vi "Autonomous IndependentAPRIL6TH (1).vi"() -> ()   [LabVIEW 2016]
doc: "This VI is called when autonomous begins, and will automatically be terminated when autonomous ends. You can carry out timed or sensor driven robot movement independently without needing to return to the caller."
uses:
  <vilib>/Rock Robotics/WPI/Utilities/WPI_GetSetVariantRefNum.vi
  <vilib>/Rock Robotics/Network Tables/NT Read String.vi
  <vilib>/Rock Robotics/Network Tables/NT Write Numeric Array.vi
  <vilib>/Rock Robotics/WPI/RobotDrive/WPI_RobotDriveArcadeDrive_Standard(NoSaturation).vi
  <vilib>/Rock Robotics/Network Tables/NT Write Number.vi
  Robot Global Data.vi
  <vilib>/Rock Robotics/WPI/Counter/WPI_CounterDigitalInputToDigitalSource.vi
  <vilib>/Rock Robotics/SystemInterfaces/DIO/FPGA_DIOChannel.ctl
panel:
  out "Hook Center Cons":dbl
  out "gyro":dbl
  out "sonar distance (inches)":dbl
  out "Encoder Loop":dbl
  out "Encoder Loop":string
  out "Current Movement, for debugging 2":T1 {"Y Joystick Value" scale=1.0..-1.0; "X Joystick Value" scale=-1.0..1.0}
  in  "Array of robot movements 2":T2(array[cluster])=[{"X Joystick Value"=0.39393939393939403, "Y Joystick Value"=0.0, "Delay (sec)"=1.0, "Movement Name"="turn"}, {"X Joystick Value"=-0.3737373737373737, "Y Joystick Value"=0.0, "Delay (sec)"=1.0, "Movement Name"="turn back"}] {"Y Joystick Value" scale=1.0..-1.0; "X Joystick Value" scale=-1.0..1.0}
  out "Current Movement, for debugging":T1 {"Y Joystick Value" scale=1.0..-1.0; "X Joystick Value" scale=-1.0..1.0}
  in  "Array of robot movements":T2(array[cluster])=[{"X Joystick Value"=0.39393939393939403, "Y Joystick Value"=0.0, "Delay (sec)"=1.0, "Movement Name"="turn"}, {"X Joystick Value"=-0.3737373737373737, "Y Joystick Value"=0.0, "Delay (sec)"=1.0, "Movement Name"="turn back"}] {"Y Joystick Value" scale=1.0..-1.0; "X Joystick Value" scale=-1.0..1.0}
  # "Sensor Readings\nConstanly updated in\nwhile loopes"
  # "Be sure to right-click and choose Data Operations>>Make Current Value default if you want to save the array values with the VI"
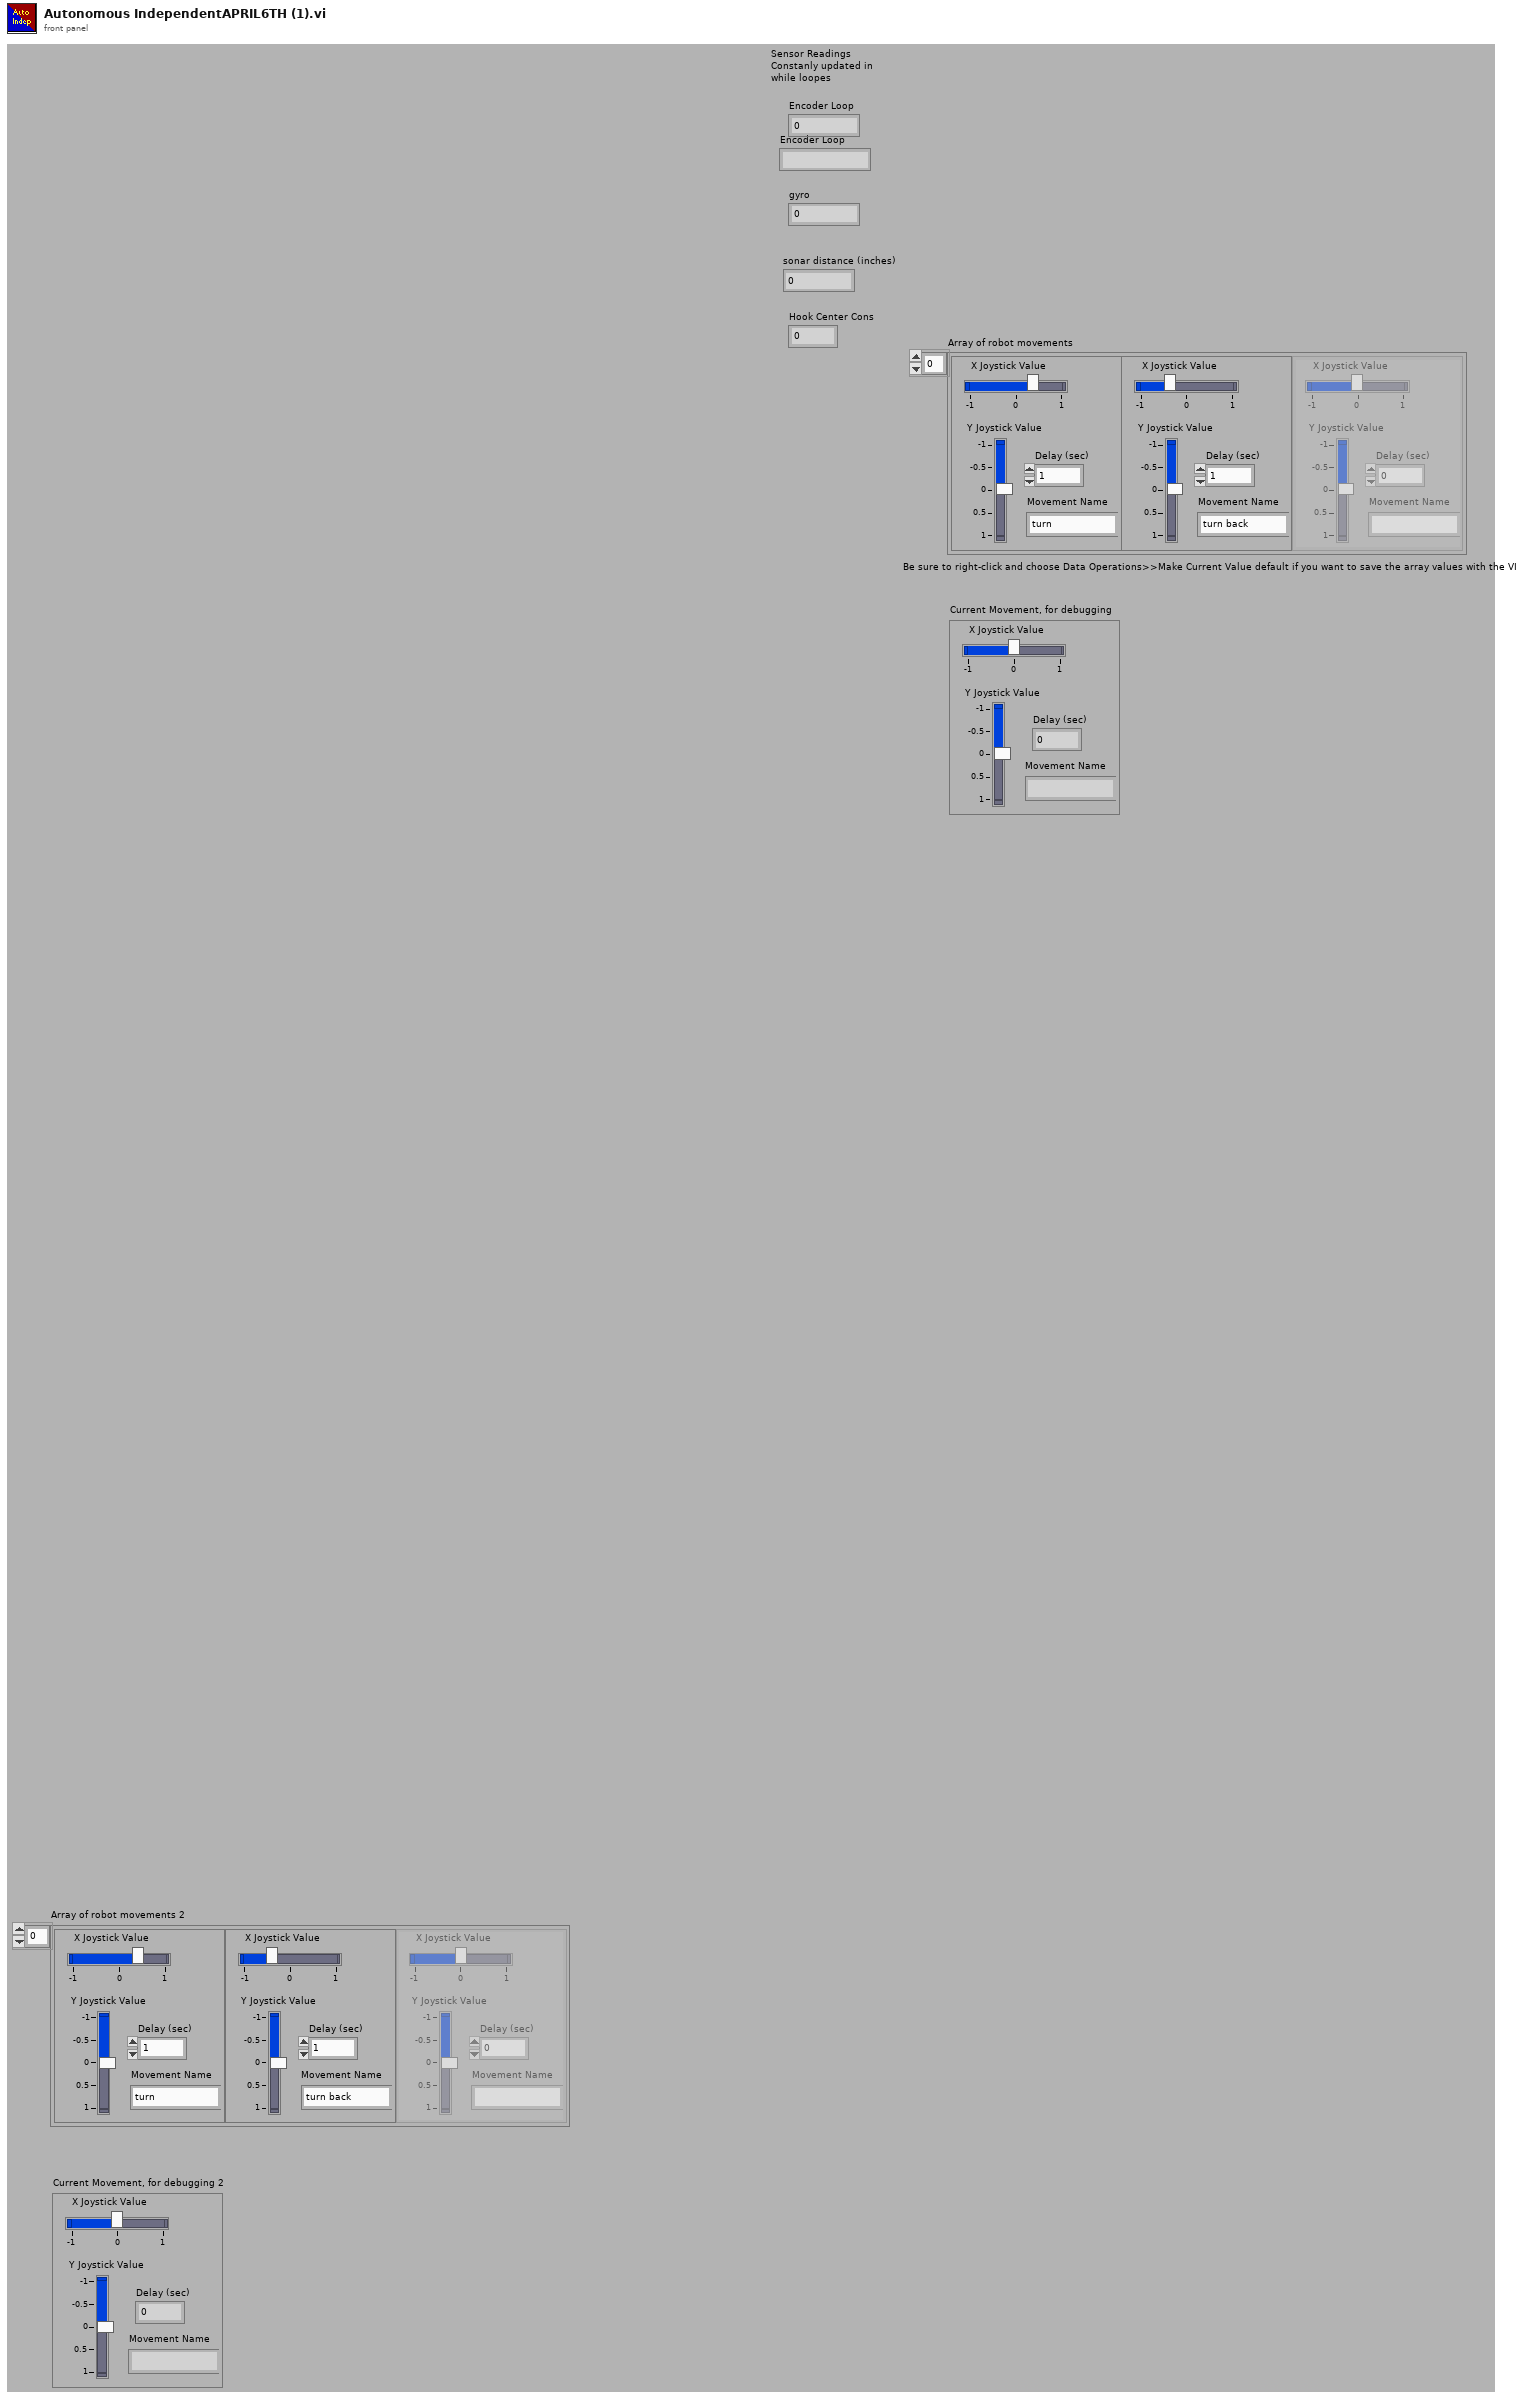
[diagram p1: front panel]
types:
  T1 = cluster{"X Joystick Value":dbl, "Y Joystick Value":dbl, "Delay (sec)":dbl, "Movement Name":string}
  T2 = cluster{"X Joystick Value":dbl, "Y Joystick Value":dbl, "Delay (sec)":dbl, "Movement Name":string}[]
  T3 = typedef "FPGA_DIOChannel.ctl" = enum8{"DIO 0", "DIO 1", "DIO 2", "DIO 3", "DIO 4", "DIO 5", "DIO 6", "DIO 7", "DIO 8", "DIO 9", "DIO MXP 0", "DIO MXP 1", "DIO MXP 2", "DIO MXP 3", "DIO MXP 4", "DIO MXP 5", "DIO MXP 6", "DIO MXP 7", "DIO MXP 8", "DIO MXP 9", "DIO MXP 10", "DIO MXP 11", "DIO MXP 12", "DIO MXP 13", "DIO MXP 14", "DIO MXP 15", "SPI Port CS1", "SPI Port CS2", "SPI Port CS3", "SPI Port MISO", "SPI Port MOSI", "Invalid"}
  T4 = typedef "WPI_DigitalInputDevRef.ctl" = cluster{"DevStatus":errorcluster, "DIO Channel":T3}
  T5 = typedef "FPGA_CounterEncoderSourceConvertionLVSourceType.ctl" = cluster{"DevStatus":errorcluster, "AnalogTriggerMode?":bool, "DigitalMode":cluster{"DIO Channel":T6}, "AnalogTriggerMode":cluster{"AnalogTriggerIndex":T7, "OutputType":T8}}
  T6 = typedef "FPGA_DIODigitalSourceChannel.ctl" = enum8{"DIO 0", "DIO 1", "DIO 2", "DIO 3", "DIO 4", "DIO 5", "DIO 6", "DIO 7", "DIO 8", "DIO 9", "DIO MXP 0", "DIO MXP 1", "DIO MXP 2", "DIO MXP 3", "DIO MXP 4", "DIO MXP 5", "DIO MXP 6", "DIO MXP 7", "DIO MXP 8", "DIO MXP 9", "DIO MXP 10", "DIO MXP 11", "DIO MXP 12", "DIO MXP 13", "DIO MXP 14", "DIO MXP 15", "Disabled"}
  T7 = typedef "FPGA_AnalogTriggerIndex.ctl" = enum8{"Trig 0", "Trig 1", "Trig 2", "Trig 3", "Trig 4", "Trig 5", "Trig 6", "Trig 7", "Invalid"}
  T8 = typedef "FPGA_AnalogTriggerOutType.ctl" = enum16{"InWindow", "TriggerState", "Rising", "Falling"}
  T9 = typedef "WPI_EncoderDevRef.ctl" = cluster{"DevStatus":errorcluster, "EncoderIndex":T10, "CounterIndex":T11, "DistancePerCount":dbl, "Decoding Type":T12}
  T10 = typedef "FPGA_EncoderIdx.ctl" = enum8{"Enc 0", "Enc 1", "Enc 2", "Enc 3", "Enc 4", "Enc 5", "Enc 6", "Enc 7", "Invalid"}
  T11 = typedef "FPGA_CounterCtrSystemIndex.ctl" = enum8{"Ctr 0", "Ctr 1", "Ctr 2", "Ctr 3", "Ctr 4", "Ctr 5", "Ctr 6", "Ctr 7", "Invalid"}
  T12 = typedef "WPI_EncoderType.ctl" = enum16{"1x", "2x", "4x"}
  T13 = typedef "WPI_JoystickDevRef.ctl" = cluster{"Device":T14}
  T14 = typedef "WPI_JoystickDeviceEnum.ctl" = enum16{"USB 0", "USB 1", "USB 2", "USB 3", "USB 4", "USB 5"}
  T15 = typedef "WPI_DriverStationPositionInfo.ctl" = enum16{"1", "2", "3"}
  T16 = typedef "WPI_RobotDriveDevRef.ctl" = cluster{"DevStatus":errorcluster, "Motors[]":T17[], "Square Inputs":bool, "Max Output":dbl}
  T17 = typedef "WPI_MotorControlDeviceRef.ctl" = cluster{"DeviceStatus":errorcluster, "Type":T18, "PWM":cluster{"PWM Channel":T19, "DeadBand":T20}, "CAN":cluster{"Device Number":u8, "SetOutput VI Ref":variant, "GetOutput VI Ref":variant, "Enable VI Ref":variant, "Disable VI Ref":variant, "Data":variant}, "Invert":bool}
  T18 = typedef "WPI_MotorControlType.ctl" = enum16{"PWM", "CAN"}
  T19 = typedef "FPGA_DIOPWMChannel.ctl" = enum8{"PWM 0", "PWM 1", "PWM 2", "PWM 3", "PWM 4", "PWM 5", "PWM 6", "PWM 7", "PWM 8", "PWM 9", "PWM MXP 0", "PWM MXP 1", "PWM MXP 2", "PWM MXP 3", "PWM MXP 4", "PWM MXP 5", "PWM MXP 6", "PWM MXP 7", "PWM MXP 8", "PWM MXP 9", "Invalid"}
  T20 = typedef "WPI_PWMDeadband.ctl" = cluster{"Name":string, "maxPositivePwm":i32, "minPositivePwm":i32, "centerPwm":i32, "maxNegativePwm":i32, "minNegativePwm":i32, "angularRange":u16}
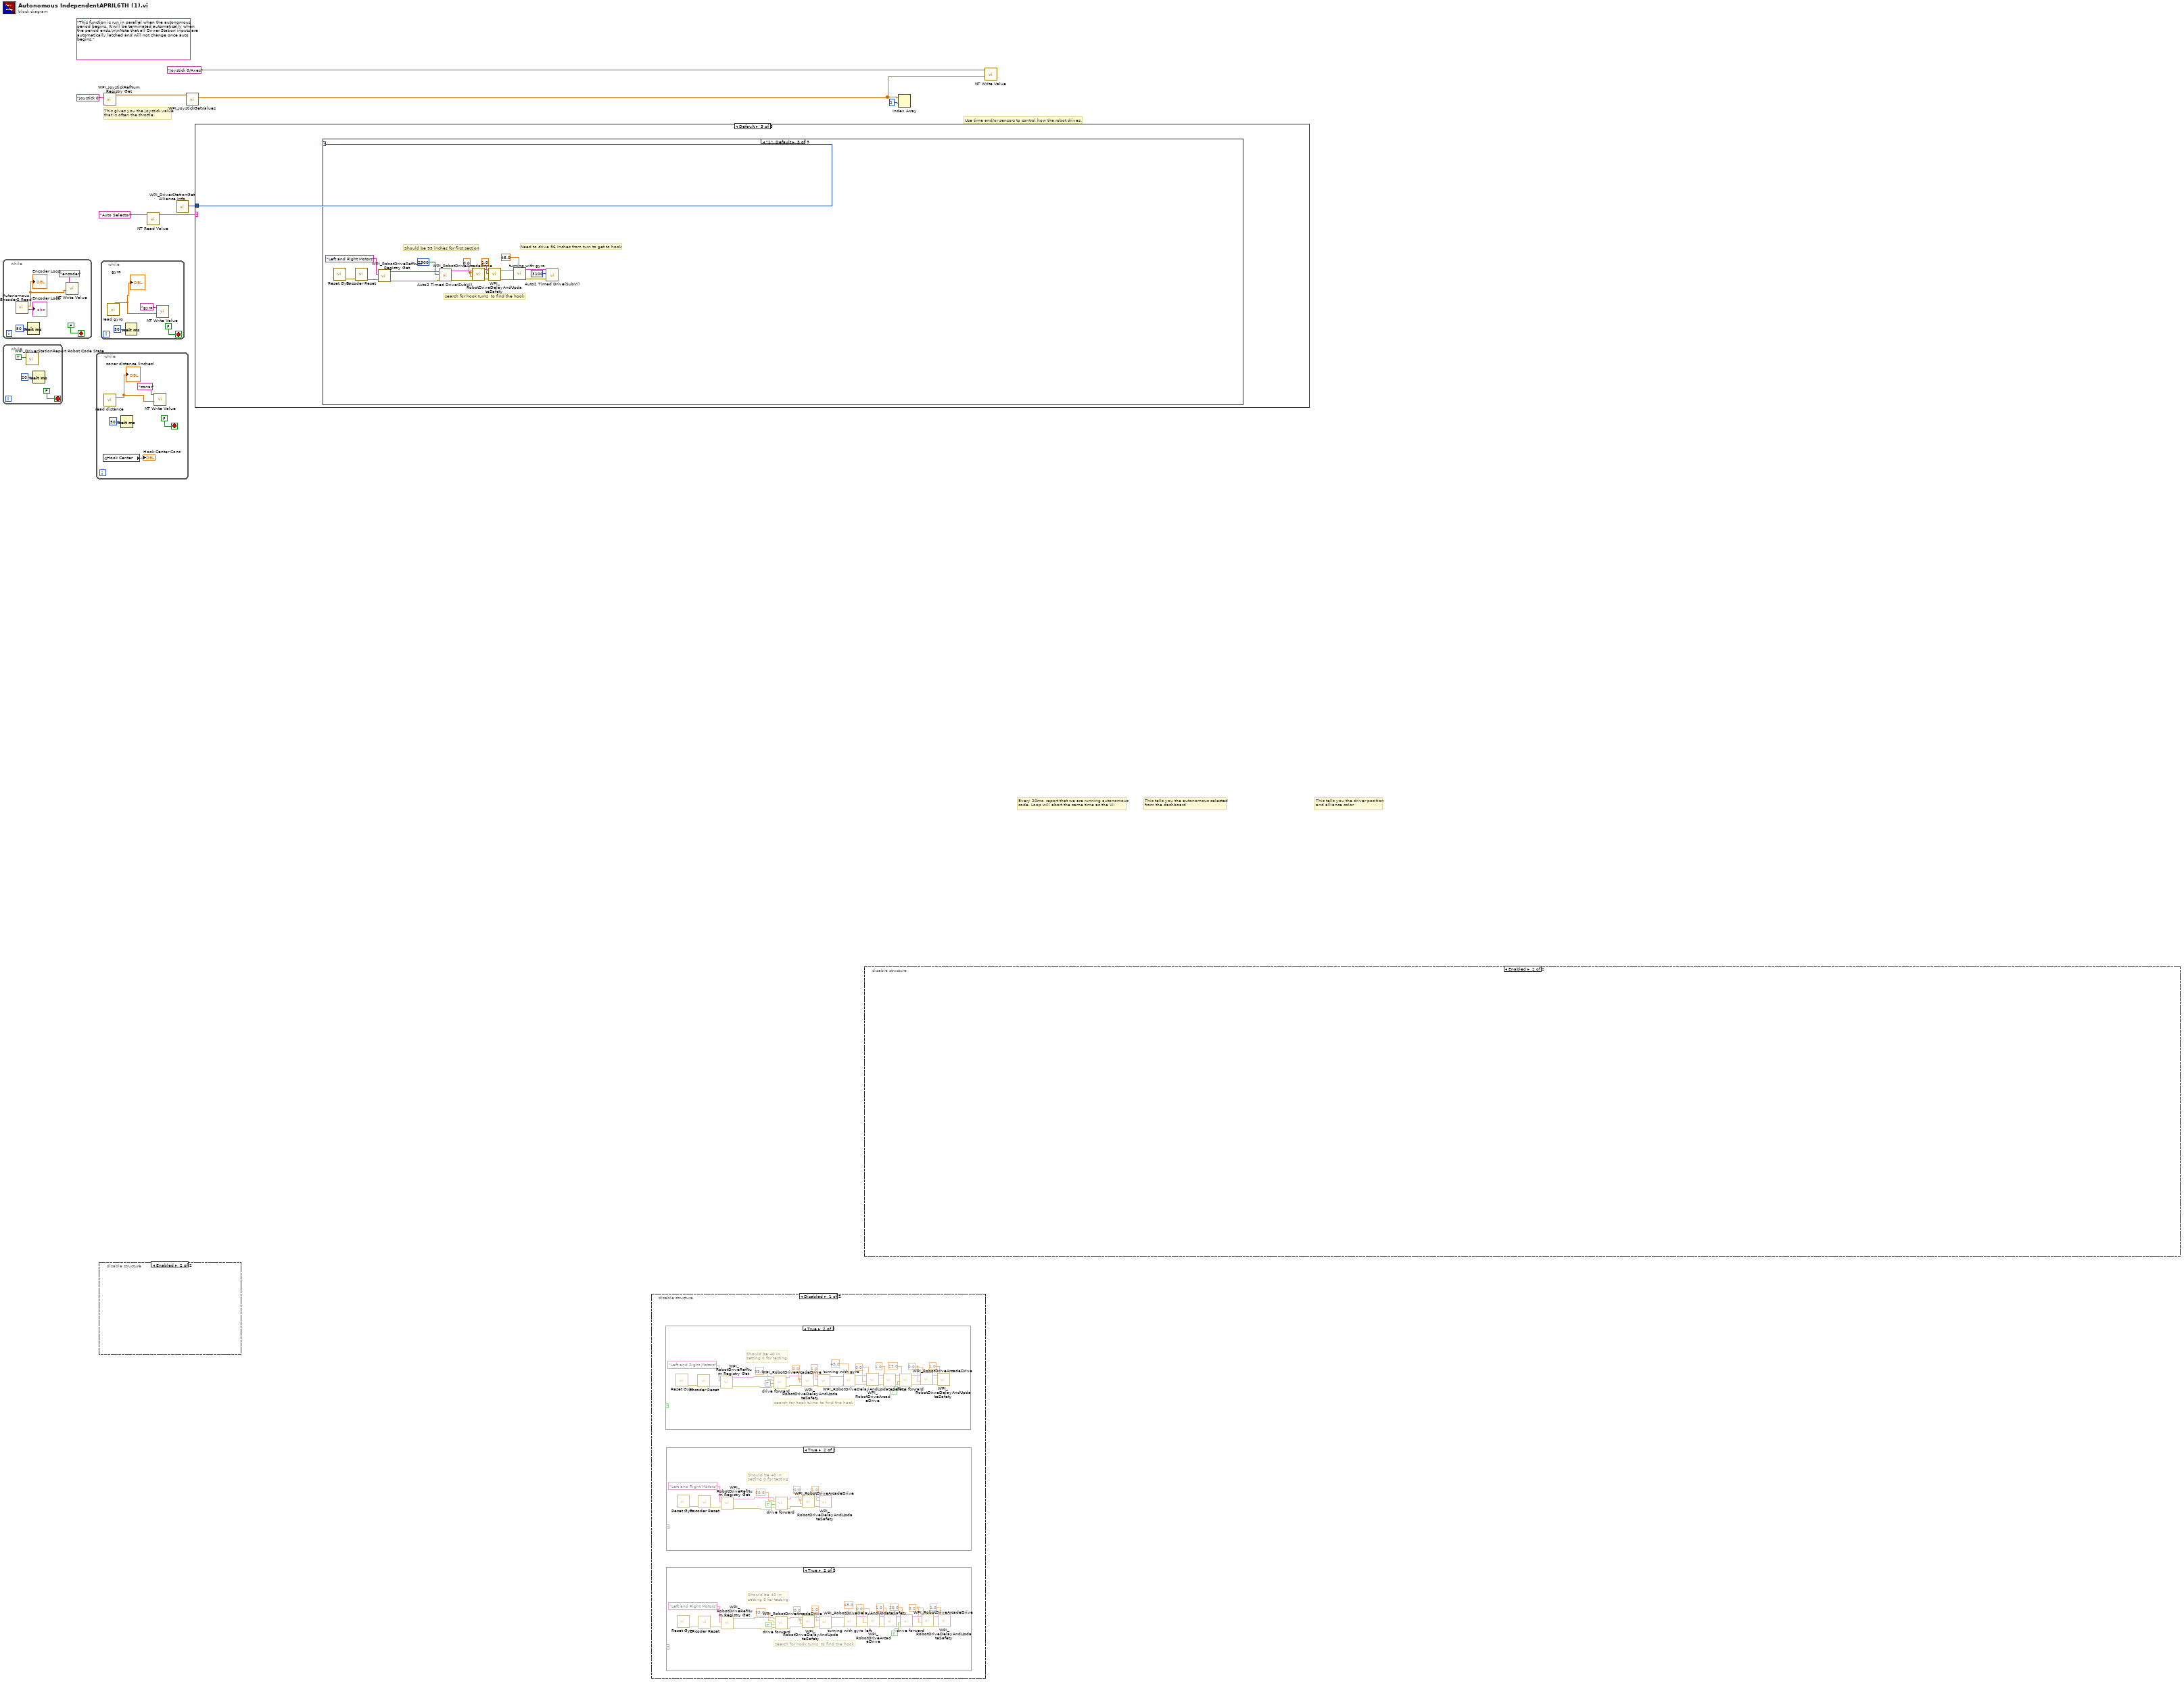
[diagram p0: block diagram]
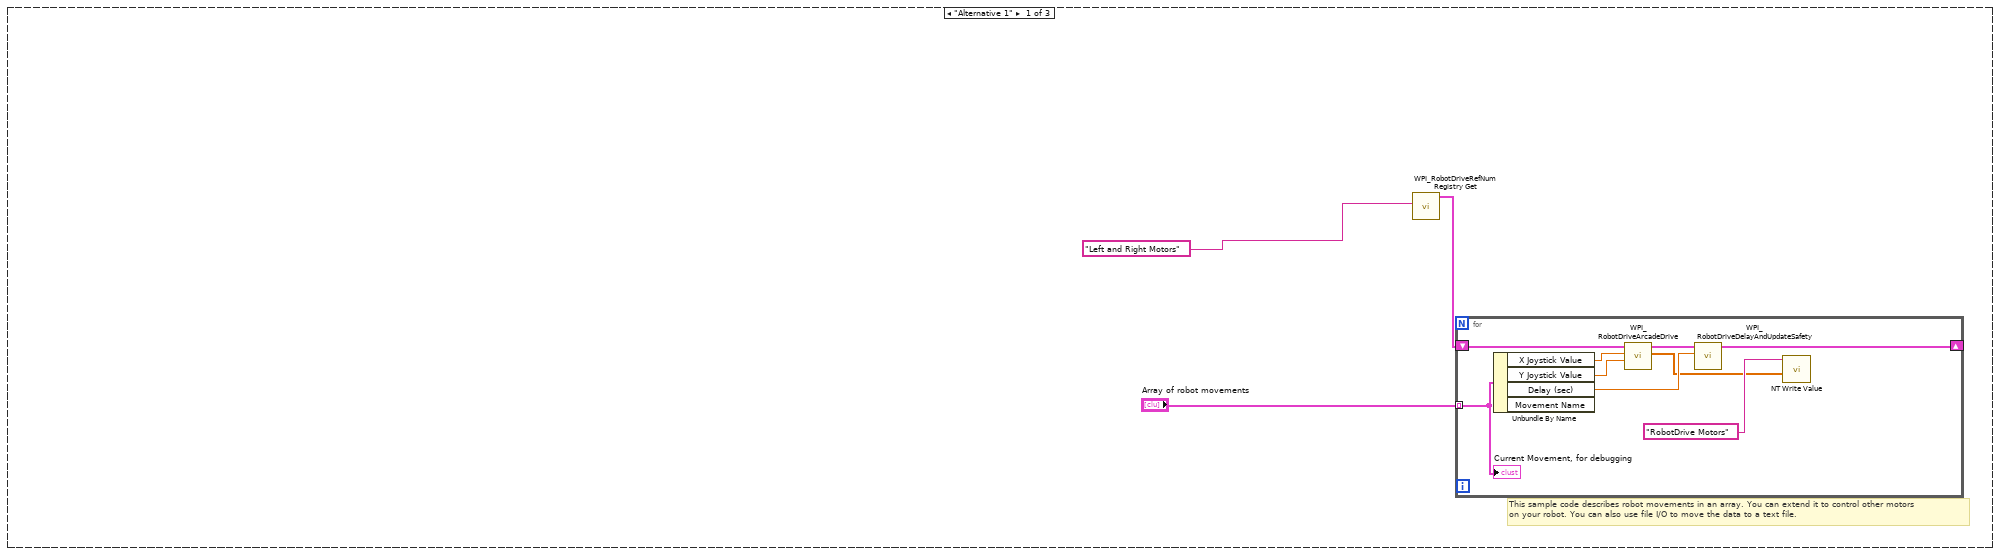
[diagram p6: hidden frame]
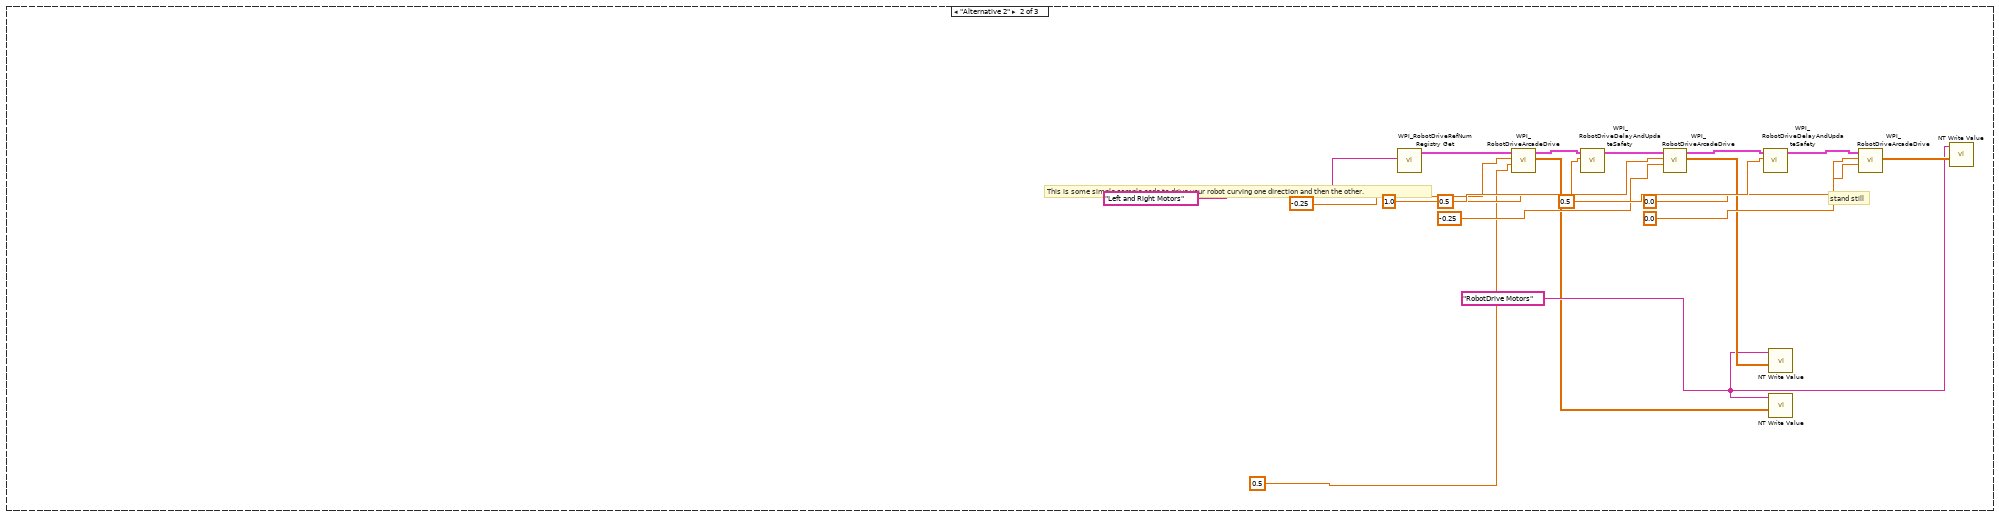
[diagram p7: hidden frame]
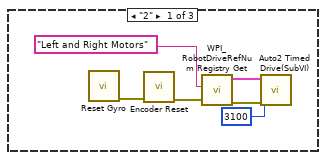
[diagram p8: hidden frame]
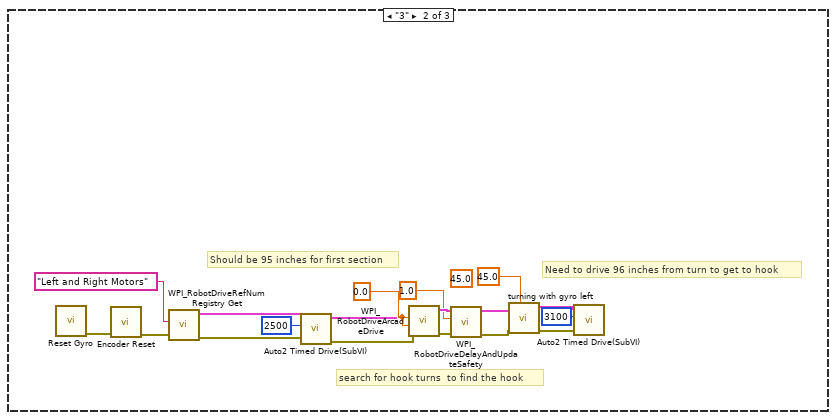
[diagram p9: hidden frame]
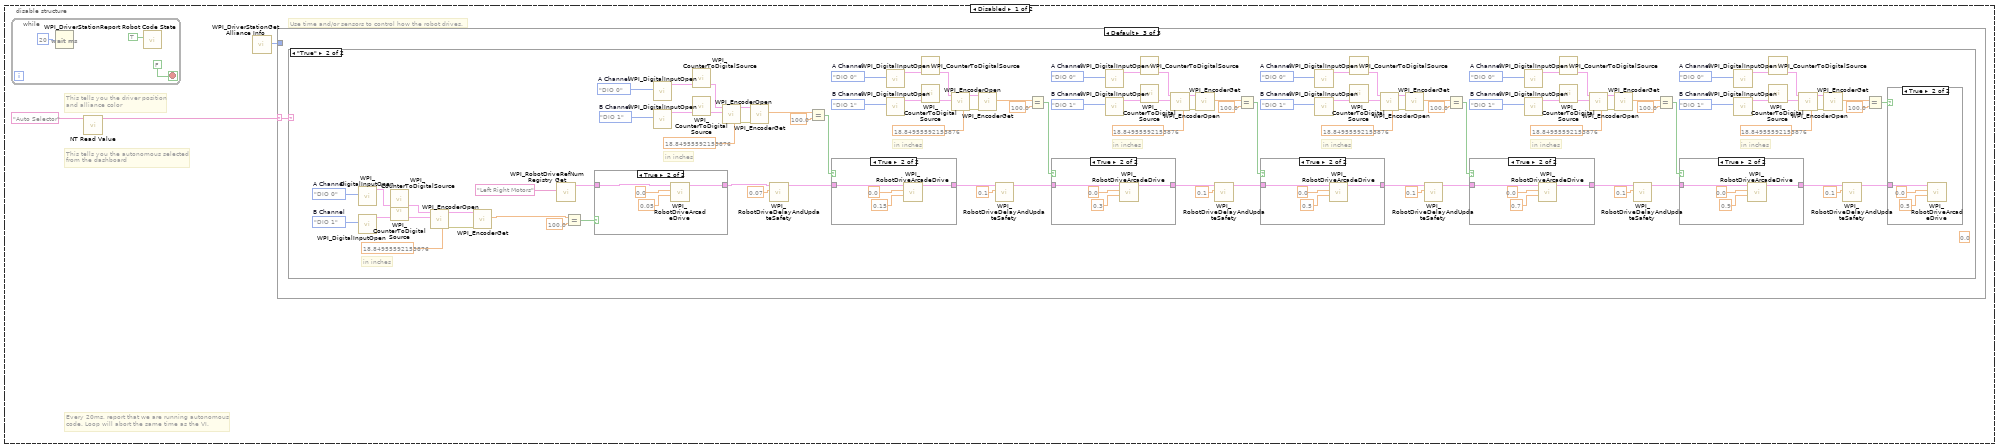
[diagram p10: hidden frame]
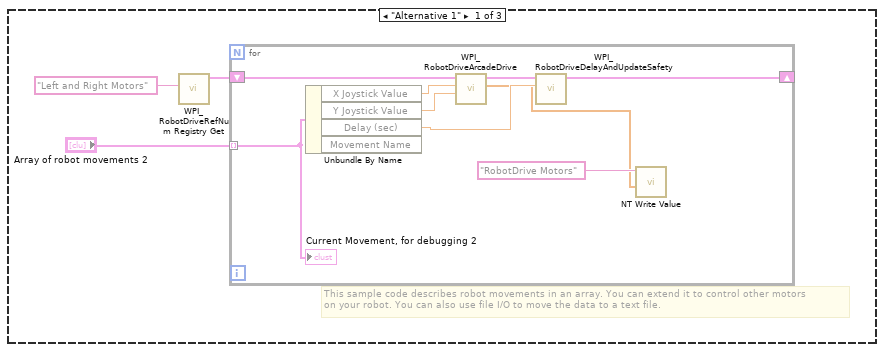
[diagram p11: hidden frame]
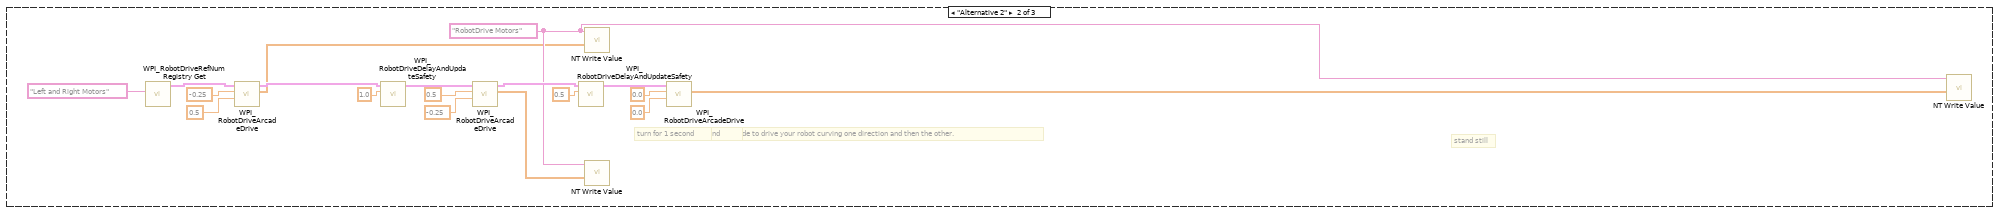
[diagram p12: hidden frame]
diagram:
  (unwired) "This function is run in parallel when the autonomous period begins. It will be terminated automatically when the period ends.\n\nNote that all Driver Station inputs are automatically latched and will not change once auto begins."
  # "This tells you the autonomous selected\nfrom the dashboard"
  # "Every 20ms, report that we are running autonomous\ncode. Loop will abort the same time as the VI."
  # "This gives you the joystick value\nthat is often the throttle"
  # "Use time and/or sensors to control how the robot drives."
  # "This tells you the driver position\nand alliance color"
  n1 = while {
    stop <- FALSE stop-if-true
    n2 = call "Autonomous Encoder2 Read.vi"() -> ("Encoder Direction"=→"Encoder Loop":string, "Encoder Distance"=w10:dbl)  [unwired: 9 in, 1 out]
    "Encoder Loop" <- w10
    n3 = Wait (ms)(milliseconds to wait=u32 50) -> ()  [unwired: 1 out]
    n4 = call-poly <vilib>:"NT Write Value.vi"("Numeric"=w10, "Name"="encoder") -> ()  [unwired: 9 in, 1 out]
  }
  n5 = while {
    stop <- FALSE stop-if-true
    n6 = call <vilib>:"WPI_DriverStationReport Robot Code State.vi"("Autonomous"=TRUE) -> ()  [unwired: 10 in, 1 out]
    n7 = Wait (ms)(milliseconds to wait=u32 20) -> ()  [unwired: 1 out]
  }
  n8 = while {
    stop <- FALSE stop-if-true
    n9 = global read "Robot Global Data.vi" "Hook Center"() -> (→"Hook Center Cons":dbl)
    n10 = call "read distance.vi"() -> ("Distance 2"=w19:dbl)  [unwired: 10 in, 1 out]
    "sonar distance (inches)" <- w19
    n11 = Wait (ms)(milliseconds to wait=u32 50) -> ()  [unwired: 1 out]
    n12 = call-poly <vilib>:"NT Write Value.vi"("Numeric"=w19, "Name"="sonar") -> ()  [unwired: 9 in, 1 out]
  }
  n13 = disable-structure shown="Enabled" {
    frame Disabled {
      w35 = FPGA_DIOChannel."DIO 1"  # B Channel
      w34 = FPGA_DIOChannel."DIO 0"  # A Channel
      # "in inches"
      n14 = call <vilib>:"WPI_DigitalInputOpen.vi"("DIO Channel"=w34) -> ("DigitalInputDevRef"=w31:T4)  [unwired: 1 in, 9 out]
      n15 = call <vilib>:"WPI_DigitalInputOpen.vi"("DIO Channel"=w35) -> ("DigitalInputDevRef"=w32:T4)  [unwired: 1 in, 9 out]
      n16 = call-poly <vilib>:"WPI_CounterToDigitalSource.vi"("DigitalInputDevRef"=w31) -> ("Digital Source"=w30:T5)  [unwired: 6 out]
      n17 = call-poly <vilib>:"WPI_CounterToDigitalSource.vi"("DigitalInputDevRef"=w32) -> ("Digital Source"=w33:T5)  [unwired: 6 out]
      n18 = call <vilib>:"WPI_EncoderOpen.vi"("DistancePerCount"=18.84955592153876, "Invert Direction (False)"=FALSE, "BSource"=w33, "ASource"=w30) -> ("error out"=w28:errorcluster, "EncoderDevRef"=w29:T9)  [unwired: 4 in, 2 out]
      n19 = call-poly <vilib>:"NT Write Value.vi"("Name"="Encoder Distance") -> ()  [unwired: 10 in, 1 out]
      n20 = call <vilib>:"WPI_EncoderRefNum Registry Set.vi"("error in (no error)"=w28, "refnum name"="Encoder", "EncoderDevRef"=w29) -> ("error out"=w26:errorcluster, "EncoderDevRef"=w27:T9)  [unwired: 7 in]
      n21 = call <vilib>:"WPI_EncoderGet.vi"("error in (no error)"=w26, "EncoderDevRef"=w27) -> ()  [unwired: 4 in, 6 out]
    }
    frame Enabled {
    }
  }
  n22 = while {
    stop <- FALSE stop-if-true
    n23 = call "read gyro.vi"() -> ("Angle 2"=w37:dbl)  [unwired: 10 in, 1 out]
    "gyro" <- w37
    n24 = Wait (ms)(milliseconds to wait=u32 50) -> ()  [unwired: 1 out]
    n25 = call-poly <vilib>:"NT Write Value.vi"("Numeric"=w37, "Name"="gyro") -> ()  [unwired: 9 in, 1 out]
  }
  n26 = call <vilib>:"WPI_JoystickRefNum Registry Get.vi"("refnum name"="Joystick 0") -> ("JoystickDevRef"=w7:T13)  [unwired: 1 in, 9 out]
  n27 = call-poly <vilib>:"NT Read Value.vi"("Name"="Auto Selector") -> ("String"=w4:string)  [unwired: 9 in, 1 out]
  n28 = call <vilib>:"WPI_DriverStationGet Alliance Info.vi"() -> ("Position"=w1:T15)  [unwired: 11 out]
  n29 = call <vilib>:"WPI_JoystickGetValues.vi"("JoystickDevRef"=w7) -> ("Axes"=w3:dbl[])  [unwired: 6 in, 4 out]
  n30 = case shown="Default" w4 {
    tunnel: w1 -> [_ _ w70]
    frame "Alternative 1" {
      # "This sample code describes robot movements in an array. You can extend it to control other motors\non your robot. You can also use file I/O to move the data to a text file."
      n31 = call <vilib>:"WPI_RobotDriveRefNum Registry Get.vi"("refnum name"="Left and Right Motors") -> ("RobotDriveDevRef"=w41:T16)  [unwired: 1 in, 9 out]
      n32 = for {
        shift-right: [w49] -> _
        shift-left: w41 -> [w50]
        tunnel: "Array of robot movements" -> [w45] mode=indexing
        n33 = Unbundle By Name(w45) -> ("X Joystick Value"=w48:dbl, "Y Joystick Value"=w47:dbl, "Delay (sec)"=w46:dbl)  [unwired: 1 out]
        n34 = call-poly <vilib>:"WPI_RobotDriveArcadeDrive.vi"("Y axis value"=w47, "X axis value"=w48, "RobotDriveDevRef"=w50) -> ("Motor Values"=w43:dbl[], "RobotDriveDevRef"=w51:T16)  [unwired: 1 in, 6 out]
        n35 = call <vilib>:"WPI_RobotDriveDelayAndUpdateSafety.vi"("Delay (s)"=w46, "RobotDriveDevRef"=w51) -> ("RobotDriveDevRef 2"=w49:T16)  [unwired: 8 in, 1 out]
        n36 = call-poly <vilib>:"NT Write Value.vi"("Numeric Array"=w43, "Name"="RobotDrive Motors") -> ()  [unwired: 9 in, 1 out]
        "Current Movement, for debugging" <- w45
      }
    }
    frame "Alternative 2" {
      w53 = "RobotDrive Motors" ("Name")
      # "This is some simple sample code to drive your robot curving one direction and then the other."
      # "stand still"
      n37 = call <vilib>:"WPI_RobotDriveRefNum Registry Get.vi"("refnum name"="Left and Right Motors") -> ("RobotDriveDevRef"=w69:T16)  [unwired: 1 in, 9 out]
      n38 = call-poly <vilib>:"WPI_RobotDriveArcadeDrive.vi"("Y axis value"=0.5 ("X axis value"), "X axis value"=-0.25, "RobotDriveDevRef"=w69) -> ("Motor Values"=w52:dbl[], "RobotDriveDevRef"=w62:T16)  [unwired: 1 in, 6 out]
      n39 = call <vilib>:"WPI_RobotDriveDelayAndUpdateSafety.vi"("Delay (s)"=1.0, "RobotDriveDevRef"=w62) -> ("RobotDriveDevRef 2"=w63:T16)  [unwired: 8 in, 1 out]
      n40 = call-poly <vilib>:"WPI_RobotDriveArcadeDrive.vi"("Y axis value"=-0.25 ("X axis value"), "X axis value"=0.5, "RobotDriveDevRef"=w63) -> ("Motor Values"=w54:dbl[], "RobotDriveDevRef"=w64:T16)  [unwired: 1 in, 6 out]
      n41 = call <vilib>:"WPI_RobotDriveDelayAndUpdateSafety.vi"("Delay (s)"=0.5, "RobotDriveDevRef"=w64) -> ("RobotDriveDevRef 2"=w65:T16)  [unwired: 8 in, 1 out]
      n42 = call-poly <vilib>:"NT Write Value.vi"("Numeric Array"=w54, "Name"=w53) -> ()  [unwired: 9 in, 1 out]
      n43 = call-poly <vilib>:"NT Write Value.vi"("Numeric Array"=w52, "Name"=w53) -> ()  [unwired: 9 in, 1 out]
      n44 = call-poly <vilib>:"WPI_RobotDriveArcadeDrive.vi"("Y axis value"=0.0 ("X axis value"), "X axis value"=0.0, "RobotDriveDevRef"=w65) -> ("Motor Values"=w55:dbl[])  [unwired: 1 in, 7 out]
      n45 = call-poly <vilib>:"NT Write Value.vi"("Numeric Array"=w55, "Name"=w53) -> ()  [unwired: 9 in, 1 out]
    }
    frame Default {
      n46 = case shown="\"1\", Default" w70 {
        frame "2" {
          n47 = call "Reset Gyro.vi"() -> ("error out"=w74:errorcluster)  [unwired: 11 in]
          n48 = call "Encoder Reset.vi"("error in (no error)"=w74) -> ("error out"=w75:errorcluster)  [unwired: 10 in]
          n49 = call <vilib>:"WPI_RobotDriveRefNum Registry Get.vi"("error in (no error)"=w75, "refnum name"="Left and Right Motors") -> ("error out"=w72:errorcluster, "RobotDriveDevRef"=w73:T16)  [unwired: 8 out]
          n50 = call "Auto2 Timed Drive(SubVI).vi"("error in (no error)"=w72, "milliseconds to wait"=u32 3100, "RobotDriveDevRef in"=w73) -> ()  [unwired: 7 in, 2 out]
        }
        frame "3" {
          (unwired) 45.0 ("desired angle")
          w88 = 0.0 ("X axis value")
          # "Should be 95 inches for first section"
          # "Need to drive 96 inches from turn to get to hook"
          # "search for hook turns  to find the hook"
          n51 = call "Reset Gyro.vi"() -> ("error out"=w92:errorcluster)  [unwired: 11 in]
          n52 = call "Encoder Reset.vi"("error in (no error)"=w92) -> ("error out"=w93:errorcluster)  [unwired: 10 in]
          n53 = call <vilib>:"WPI_RobotDriveRefNum Registry Get.vi"("error in (no error)"=w93, "refnum name"="Left and Right Motors") -> ("error out"=w86:errorcluster, "RobotDriveDevRef"=w87:T16)  [unwired: 8 out]
          n54 = call "Auto2 Timed Drive(SubVI).vi"("error in (no error)"=w86, "milliseconds to wait"=u32 2500, "RobotDriveDevRef in"=w87) -> ("error out"=w84:errorcluster, "RobotDriveDevRef out"=w85:T16)  [unwired: 7 in]
          n55 = call-poly <vilib>:"WPI_RobotDriveArcadeDrive.vi"("error in (no error)"=w84, "Y axis value"=w88, "X axis value"=w88, "RobotDriveDevRef"=w85) -> ("error out"=w90:errorcluster, "RobotDriveDevRef"=w91:T16)  [unwired: 6 out]
          n56 = call <vilib>:"WPI_RobotDriveDelayAndUpdateSafety.vi"("error in (no error)"=w90, "Delay (s)"=1.0, "RobotDriveDevRef"=w91) -> ("error out"=w81:errorcluster, "RobotDriveDevRef 2"=w82:T16)  [unwired: 7 in]
          n57 = call "turning with gyro left.vi"("desired angle"=45.0, "error in (no error)"=w81, "RobotDriveDevRef"=w82) -> ("error out"=w78:errorcluster, "RobotDriveDevRef 2"=w79:T16)  [unwired: 6 in, 1 out]
          n58 = call "Auto2 Timed Drive(SubVI).vi"("error in (no error)"=w78, "milliseconds to wait"=u32 3100, "RobotDriveDevRef in"=w79) -> ()  [unwired: 7 in, 2 out]
        }
        frame "1", Default {
          w106 = 0.0 ("X axis value")
          # "Need to drive 96 inches from turn to get to hook"
          # "search for hook turns  to find the hook"
          # "Should be 95 inches for first section"
          n59 = call "Reset Gyro.vi"() -> ("error out"=w110:errorcluster)  [unwired: 11 in]
          n60 = call "Encoder Reset.vi"("error in (no error)"=w110) -> ("error out"=w111:errorcluster)  [unwired: 10 in]
          n61 = call <vilib>:"WPI_RobotDriveRefNum Registry Get.vi"("error in (no error)"=w111, "refnum name"="Left and Right Motors") -> ("error out"=w101:errorcluster, "RobotDriveDevRef"=w102:T16)  [unwired: 8 out]
          n62 = call "Auto2 Timed Drive(SubVI).vi"("error in (no error)"=w101, "milliseconds to wait"=u32 2500, "RobotDriveDevRef in"=w102) -> ("error out"=w99:errorcluster, "RobotDriveDevRef out"=w100:T16)  [unwired: 7 in]
          n63 = call-poly <vilib>:"WPI_RobotDriveArcadeDrive.vi"("error in (no error)"=w99, "Y axis value"=w106, "X axis value"=w106, "RobotDriveDevRef"=w100) -> ("error out"=w108:errorcluster, "RobotDriveDevRef"=w109:T16)  [unwired: 6 out]
          n64 = call <vilib>:"WPI_RobotDriveDelayAndUpdateSafety.vi"("error in (no error)"=w108, "Delay (s)"=1.0, "RobotDriveDevRef"=w109) -> ("error out"=w104:errorcluster, "RobotDriveDevRef 2"=w105:T16)  [unwired: 7 in]
          n65 = call "turning with gyro.vi"("desired angle"=45.0, "error in (no error)"=w104, "RobotDriveDevRef"=w105) -> ("error out"=w96:errorcluster, "RobotDriveDevRef 2"=w97:T16)  [unwired: 7 in]
          n66 = call "Auto2 Timed Drive(SubVI).vi"("error in (no error)"=w96, "milliseconds to wait"=u32 3100, "RobotDriveDevRef in"=w97) -> ()  [unwired: 7 in, 2 out]
        }
      }
    }
  }
  n67 = disable-structure shown="Disabled" {
    frame Disabled {
      n68 = case shown="True" {
        selector: _ -> [_ _]
        frame False {
        }
        frame True {
          w161 = 0.0 ("X axis value")
          w172 = 0.0 ("X axis value")
          w179 = 0.0 ("X axis value")
          # "search for hook turns  to find the hook"
          # "Should be 40 in\nsetting 0 for testing"
          n69 = call "Reset Gyro.vi"() -> ("error out"=w186:errorcluster)  [unwired: 11 in]
          n70 = call "Encoder Reset.vi"("error in (no error)"=w186) -> ("error out"=w188:errorcluster)  [unwired: 10 in]
          n71 = call <vilib>:"WPI_RobotDriveRefNum Registry Get.vi"("error in (no error)"=w188, "refnum name"="Left and Right Motors") -> ("error out"=w185:errorcluster, "RobotDriveDevRef"=w187:T16)  [unwired: 8 out]
          n72 = call "drive forward.vi"("error in (no error)"=w185, "forward"=TRUE, "desired distance"=95.0, "RobotDriveDevRef in"=w187) -> ("error out"=w177:errorcluster, "RobotDriveDevRef out"=w178:T16)  [unwired: 6 in]
          n73 = call-poly <vilib>:"WPI_RobotDriveArcadeDrive.vi"("error in (no error)"=w177, "Y axis value"=w179, "X axis value"=w179, "RobotDriveDevRef"=w178) -> ("error out"=w181:errorcluster, "RobotDriveDevRef"=w182:T16)  [unwired: 6 out]
          n74 = call <vilib>:"WPI_RobotDriveDelayAndUpdateSafety.vi"("error in (no error)"=w181, "Delay (s)"=1.0, "RobotDriveDevRef"=w182) -> ("error out"=w175:errorcluster, "RobotDriveDevRef 2"=w176:T16)  [unwired: 7 in]
          n75 = call "turning with gyro.vi"("desired angle"=45.0, "error in (no error)"=w175, "RobotDriveDevRef"=w176) -> ("error out"=w169:errorcluster, "RobotDriveDevRef 2"=w173:T16)  [unwired: 7 in]
          n76 = call-poly <vilib>:"WPI_RobotDriveArcadeDrive.vi"("error in (no error)"=w169, "Y axis value"=w172, "X axis value"=w172, "RobotDriveDevRef"=w173) -> ("error out"=w170:errorcluster, "RobotDriveDevRef"=w171:T16)  [unwired: 6 out]
          n77 = call <vilib>:"WPI_RobotDriveDelayAndUpdateSafety.vi"("error in (no error)"=w170, "Delay (s)"=1.0, "RobotDriveDevRef"=w171) -> ("error out"=w167:errorcluster, "RobotDriveDevRef 2"=w166:T16)  [unwired: 7 in]
          n78 = call "drive forward.vi"("error in (no error)"=w167, "forward"=TRUE, "desired distance"=25.0, "RobotDriveDevRef in"=w166) -> ("error out"=w162:errorcluster, "RobotDriveDevRef out"=w163:T16)  [unwired: 6 in]
          n79 = call-poly <vilib>:"WPI_RobotDriveArcadeDrive.vi"("error in (no error)"=w162, "Y axis value"=w161, "X axis value"=w161, "RobotDriveDevRef"=w163) -> ("error out"=w159:errorcluster, "RobotDriveDevRef"=w160:T16)  [unwired: 6 out]
          n80 = call <vilib>:"WPI_RobotDriveDelayAndUpdateSafety.vi"("error in (no error)"=w159, "Delay (s)"=1.0, "RobotDriveDevRef"=w160) -> ()  [unwired: 7 in, 2 out]
        }
      }
      n81 = case shown="True" {
        selector: _ -> [_ _]
        frame False {
        }
        frame True {
          w147 = 0.0 ("X axis value")
          # "Should be 40 in\nsetting 0 for testing"
          n82 = call "Reset Gyro.vi"() -> ("error out"=w154:errorcluster)  [unwired: 11 in]
          n83 = call "Encoder Reset.vi"("error in (no error)"=w154) -> ("error out"=w156:errorcluster)  [unwired: 10 in]
          n84 = call <vilib>:"WPI_RobotDriveRefNum Registry Get.vi"("error in (no error)"=w156, "refnum name"="Left and Right Motors") -> ("error out"=w153:errorcluster, "RobotDriveDevRef"=w155:T16)  [unwired: 8 out]
          n85 = call "drive forward.vi"("error in (no error)"=w153, "forward"=TRUE, "desired distance"=60.0, "RobotDriveDevRef in"=w155) -> ("error out"=w145:errorcluster, "RobotDriveDevRef out"=w146:T16)  [unwired: 6 in]
          n86 = call-poly <vilib>:"WPI_RobotDriveArcadeDrive.vi"("error in (no error)"=w145, "Y axis value"=w147, "X axis value"=w147, "RobotDriveDevRef"=w146) -> ("error out"=w149:errorcluster, "RobotDriveDevRef"=w150:T16)  [unwired: 6 out]
          n87 = call <vilib>:"WPI_RobotDriveDelayAndUpdateSafety.vi"("error in (no error)"=w149, "Delay (s)"=1.0, "RobotDriveDevRef"=w150) -> ()  [unwired: 7 in, 2 out]
        }
      }
      n88 = case shown="True" {
        selector: _ -> [_ _]
        frame False {
        }
        frame True {
          w116 = 0.0 ("X axis value")
          w127 = 0.0 ("X axis value")
          w134 = 0.0 ("X axis value")
          # "search for hook turns  to find the hook"
          # "Should be 40 in\nsetting 0 for testing"
          n89 = call "Reset Gyro.vi"() -> ("error out"=w141:errorcluster)  [unwired: 11 in]
          n90 = call "Encoder Reset.vi"("error in (no error)"=w141) -> ("error out"=w143:errorcluster)  [unwired: 10 in]
          n91 = call <vilib>:"WPI_RobotDriveRefNum Registry Get.vi"("error in (no error)"=w143, "refnum name"="Left and Right Motors") -> ("error out"=w140:errorcluster, "RobotDriveDevRef"=w142:T16)  [unwired: 8 out]
          n92 = call "drive forward.vi"("error in (no error)"=w140, "forward"=TRUE, "desired distance"=95.0, "RobotDriveDevRef in"=w142) -> ("error out"=w132:errorcluster, "RobotDriveDevRef out"=w133:T16)  [unwired: 6 in]
          n93 = call-poly <vilib>:"WPI_RobotDriveArcadeDrive.vi"("error in (no error)"=w132, "Y axis value"=w134, "X axis value"=w134, "RobotDriveDevRef"=w133) -> ("error out"=w136:errorcluster, "RobotDriveDevRef"=w137:T16)  [unwired: 6 out]
          n94 = call <vilib>:"WPI_RobotDriveDelayAndUpdateSafety.vi"("error in (no error)"=w136, "Delay (s)"=1.0, "RobotDriveDevRef"=w137) -> ("error out"=w130:errorcluster, "RobotDriveDevRef 2"=w131:T16)  [unwired: 7 in]
          n95 = call "turning with gyro left.vi"("desired angle"=45.0, "error in (no error)"=w130, "RobotDriveDevRef"=w131) -> ("error out"=w124:errorcluster, "RobotDriveDevRef 2"=w128:T16)  [unwired: 6 in, 1 out]
          n96 = call-poly <vilib>:"WPI_RobotDriveArcadeDrive.vi"("error in (no error)"=w124, "Y axis value"=w127, "X axis value"=w127, "RobotDriveDevRef"=w128) -> ("error out"=w125:errorcluster, "RobotDriveDevRef"=w126:T16)  [unwired: 6 out]
          n97 = call <vilib>:"WPI_RobotDriveDelayAndUpdateSafety.vi"("error in (no error)"=w125, "Delay (s)"=1.0, "RobotDriveDevRef"=w126) -> ("error out"=w122:errorcluster, "RobotDriveDevRef 2"=w121:T16)  [unwired: 7 in]
          n98 = call "drive forward.vi"("error in (no error)"=w122, "forward"=TRUE, "desired distance"=25.0, "RobotDriveDevRef in"=w121) -> ("error out"=w117:errorcluster, "RobotDriveDevRef out"=w118:T16)  [unwired: 6 in]
          n99 = call-poly <vilib>:"WPI_RobotDriveArcadeDrive.vi"("error in (no error)"=w117, "Y axis value"=w116, "X axis value"=w116, "RobotDriveDevRef"=w118) -> ("error out"=w114:errorcluster, "RobotDriveDevRef"=w115:T16)  [unwired: 6 out]
          n100 = call <vilib>:"WPI_RobotDriveDelayAndUpdateSafety.vi"("error in (no error)"=w114, "Delay (s)"=1.0, "RobotDriveDevRef"=w115) -> ()  [unwired: 7 in, 2 out]
        }
      }
    }
    frame Enabled {
    }
  }
  n101 = disable-structure shown="Enabled" {
    frame Disabled {
      # "This tells you the autonomous selected\nfrom the dashboard"
      # "Every 20ms, report that we are running autonomous\ncode. Loop will abort the same time as the VI."
      # "Use time and/or sensors to control how the robot drives."
      # "This tells you the driver position\nand alliance color"
      n102 = while {
        stop <- FALSE stop-if-true
        n103 = Wait (ms)(milliseconds to wait=u32 20) -> ()  [unwired: 1 out]
        n104 = call <vilib>:"WPI_DriverStationReport Robot Code State.vi"("Autonomous"=TRUE) -> ()  [unwired: 10 in, 1 out]
      }
      n105 = call-poly <vilib>:"NT Read Value.vi"("Name"="Auto Selector") -> ("String"=w192:string)  [unwired: 9 in, 1 out]
      n106 = call <vilib>:"WPI_DriverStationGet Alliance Info.vi"() -> ("Position"=w191:T15)  [unwired: 11 out]
      n107 = case shown="Default" w192 {
        selector: w192 -> [_ _ w223]
        tunnel: w191 -> [_ _ _]
        frame "Alternative 1" {
          # "This sample code describes robot movements in an array. You can extend it to control other motors\non your robot. You can also use file I/O to move the data to a text file."
          n108 = call <vilib>:"WPI_RobotDriveRefNum Registry Get.vi"("refnum name"="Left and Right Motors") -> ("RobotDriveDevRef"=w194:T16)  [unwired: 1 in, 9 out]
          n109 = for {
            shift-right: [w202] -> _
            shift-left: w194 -> [w203]
            tunnel: "Array of robot movements 2" -> [w198] mode=indexing
            n110 = Unbundle By Name(w198) -> ("X Joystick Value"=w201:dbl, "Y Joystick Value"=w200:dbl, "Delay (sec)"=w199:dbl)  [unwired: 1 out]
            n111 = call-poly <vilib>:"WPI_RobotDriveArcadeDrive.vi"("Y axis value"=w200, "X axis value"=w201, "RobotDriveDevRef"=w203) -> ("Motor Values"=w196:dbl[], "RobotDriveDevRef"=w204:T16)  [unwired: 1 in, 6 out]
            n112 = call <vilib>:"WPI_RobotDriveDelayAndUpdateSafety.vi"("Delay (s)"=w199, "RobotDriveDevRef"=w204) -> ("RobotDriveDevRef 2"=w202:T16)  [unwired: 8 in, 1 out]
            n113 = call-poly <vilib>:"NT Write Value.vi"("Numeric Array"=w196, "Name"="RobotDrive Motors") -> ()  [unwired: 9 in, 1 out]
            "Current Movement, for debugging 2" <- w198
          }
        }
        frame "Alternative 2" {
          w206 = "RobotDrive Motors" ("Name")
          # "This is some simple sample code to drive your robot curving one direction and then the other."
          # "stand still"
          # "other way for 0.5 second"
          # "turn for 1 second"
          n114 = call <vilib>:"WPI_RobotDriveRefNum Registry Get.vi"("refnum name"="Left and Right Motors") -> ("RobotDriveDevRef"=w222:T16)  [unwired: 1 in, 9 out]
          n115 = call-poly <vilib>:"WPI_RobotDriveArcadeDrive.vi"("Y axis value"=0.5 ("X axis value"), "X axis value"=-0.25, "RobotDriveDevRef"=w222) -> ("Motor Values"=w205:dbl[], "RobotDriveDevRef"=w215:T16)  [unwired: 1 in, 6 out]
          n116 = call <vilib>:"WPI_RobotDriveDelayAndUpdateSafety.vi"("Delay (s)"=1.0, "RobotDriveDevRef"=w215) -> ("RobotDriveDevRef 2"=w216:T16)  [unwired: 8 in, 1 out]
          n117 = call-poly <vilib>:"WPI_RobotDriveArcadeDrive.vi"("Y axis value"=-0.25 ("X axis value"), "X axis value"=0.5, "RobotDriveDevRef"=w216) -> ("Motor Values"=w207:dbl[], "RobotDriveDevRef"=w217:T16)  [unwired: 1 in, 6 out]
          n118 = call <vilib>:"WPI_RobotDriveDelayAndUpdateSafety.vi"("Delay (s)"=0.5, "RobotDriveDevRef"=w217) -> ("RobotDriveDevRef 2"=w218:T16)  [unwired: 8 in, 1 out]
          n119 = call-poly <vilib>:"NT Write Value.vi"("Numeric Array"=w205, "Name"=w206) -> ()  [unwired: 9 in, 1 out]
          n120 = call-poly <vilib>:"NT Write Value.vi"("Numeric Array"=w207, "Name"=w206) -> ()  [unwired: 9 in, 1 out]
          n121 = call-poly <vilib>:"WPI_RobotDriveArcadeDrive.vi"("Y axis value"=0.0 ("X axis value"), "X axis value"=0.0, "RobotDriveDevRef"=w218) -> ("Motor Values"=w208:dbl[])  [unwired: 1 in, 7 out]
          n122 = call-poly <vilib>:"NT Write Value.vi"("Numeric Array"=w208, "Name"=w206) -> ()  [unwired: 9 in, 1 out]
        }
        frame Default {
          n123 = case shown="\"True\"" w223 {
            frame "False", Default {
            }
            frame "True" {
              w236 = FPGA_DIOChannel."DIO 1"  # B Channel
              w235 = FPGA_DIOChannel."DIO 0"  # A Channel
              w249 = FPGA_DIOChannel."DIO 1"  # B Channel
              w248 = FPGA_DIOChannel."DIO 0"  # A Channel
              w260 = FPGA_DIOChannel."DIO 1"  # B Channel
              w259 = FPGA_DIOChannel."DIO 0"  # A Channel
              w272 = FPGA_DIOChannel."DIO 1"  # B Channel
              w271 = FPGA_DIOChannel."DIO 0"  # A Channel
              w284 = FPGA_DIOChannel."DIO 1"  # B Channel
              w283 = FPGA_DIOChannel."DIO 0"  # A Channel
              w296 = FPGA_DIOChannel."DIO 1"  # B Channel
              w295 = FPGA_DIOChannel."DIO 0"  # A Channel
              w307 = FPGA_DIOChannel."DIO 1"  # B Channel
              w306 = FPGA_DIOChannel."DIO 0"  # A Channel
              (unwired) 0.0 ("Distance")
              # "in inches"
              # "in inches"
              # "in inches"
              # "in inches"
              # "in inches"
              # "in inches"
              # "in inches"
              n124 = call <vilib>:"WPI_DigitalInputOpen.vi"("DIO Channel"=w306) -> ("DigitalInputDevRef"=w303:T4)  [unwired: 1 in, 9 out]
              n125 = call <vilib>:"WPI_DigitalInputOpen.vi"("DIO Channel"=w307) -> ("DigitalInputDevRef"=w304:T4)  [unwired: 1 in, 9 out]
              n126 = call-poly <vilib>:"WPI_CounterToDigitalSource.vi"("DigitalInputDevRef"=w303) -> ("Digital Source"=w224:T5)  [unwired: 6 out]
              n127 = call-poly <vilib>:"WPI_CounterToDigitalSource.vi"("DigitalInputDevRef"=w304) -> ("Digital Source"=w305:T5)  [unwired: 6 out]
              n128 = call <vilib>:"WPI_EncoderOpen.vi"("DistancePerCount"=18.84955592153876, "BSource"=w305, "ASource"=w224) -> ("error out"=w300:errorcluster, "EncoderDevRef"=w301:T9)  [unwired: 5 in, 2 out]
              n129 = call <vilib>:"WPI_EncoderGet.vi"("error in (no error)"=w300, "EncoderDevRef"=w301) -> ("Distance"=w299:dbl)  [unwired: 4 in, 5 out]
              n130 = call <vilib>:"WPI_RobotDriveRefNum Registry Get.vi"("refnum name"="Left Right Motors") -> ("RobotDriveDevRef"=w326:T16)  [unwired: 9 in, 1 out]
              n131 = Equal?(x=w299, y=100.0) -> (x = y?=w297:bool)
              n132 = case shown="True" w297 {
                tunnel: w326 -> [w356 w360]
                tunnel: [w356 w357] -> w325
                frame False {
                }
                frame True {
                  n133 = call-poly <vilib>:"WPI_RobotDriveArcadeDrive.vi"("Y axis value"=0.05, "X axis value"=0.0, "RobotDriveDevRef"=w360) -> ("RobotDriveDevRef"=w357:T16)  [unwired: 6 in, 2 out]
                }
              }
              n134 = call <vilib>:"WPI_DigitalInputOpen.vi"("DIO Channel"=w295) -> ("DigitalInputDevRef"=w292:T4)  [unwired: 1 in, 9 out]
              n135 = call <vilib>:"WPI_DigitalInputOpen.vi"("DIO Channel"=w296) -> ("DigitalInputDevRef"=w293:T4)  [unwired: 1 in, 9 out]
              n136 = call-poly <vilib>:"WPI_CounterToDigitalSource.vi"("DigitalInputDevRef"=w292) -> ("Digital Source"=w291:T5)  [unwired: 6 out]
              n137 = call-poly <vilib>:"WPI_CounterToDigitalSource.vi"("DigitalInputDevRef"=w293) -> ("Digital Source"=w294:T5)  [unwired: 6 out]
              n138 = call <vilib>:"WPI_EncoderOpen.vi"("DistancePerCount"=18.84955592153876, "BSource"=w294, "ASource"=w291) -> ("error out"=w288:errorcluster, "EncoderDevRef"=w289:T9)  [unwired: 5 in, 2 out]
              n139 = call <vilib>:"WPI_EncoderGet.vi"("error in (no error)"=w288, "EncoderDevRef"=w289) -> ("Distance"=w287:dbl)  [unwired: 4 in, 5 out]
              n140 = call <vilib>:"WPI_RobotDriveDelayAndUpdateSafety.vi"("Delay (s)"=0.07, "RobotDriveDevRef"=w325) -> ("RobotDriveDevRef 2"=w321:T16)  [unwired: 8 in, 1 out]
              n141 = Equal?(x=w287, y=100.0) -> (x = y?=w285:bool)
              n142 = case shown="True" w285 {
                tunnel: w321 -> [w351 w355]
                tunnel: [w351 w352] -> w323
                frame False {
                }
                frame True {
                  n143 = call-poly <vilib>:"WPI_RobotDriveArcadeDrive.vi"("Y axis value"=0.15, "X axis value"=0.0, "RobotDriveDevRef"=w355) -> ("RobotDriveDevRef"=w352:T16)  [unwired: 6 in, 2 out]
                }
              }
              n144 = call <vilib>:"WPI_DigitalInputOpen.vi"("DIO Channel"=w283) -> ("DigitalInputDevRef"=w280:T4)  [unwired: 1 in, 9 out]
              n145 = call <vilib>:"WPI_DigitalInputOpen.vi"("DIO Channel"=w284) -> ("DigitalInputDevRef"=w281:T4)  [unwired: 1 in, 9 out]
              n146 = call-poly <vilib>:"WPI_CounterToDigitalSource.vi"("DigitalInputDevRef"=w280) -> ("Digital Source"=w279:T5)  [unwired: 6 out]
              n147 = call-poly <vilib>:"WPI_CounterToDigitalSource.vi"("DigitalInputDevRef"=w281) -> ("Digital Source"=w282:T5)  [unwired: 6 out]
              n148 = call <vilib>:"WPI_EncoderOpen.vi"("DistancePerCount"=18.84955592153876, "BSource"=w282, "ASource"=w279) -> ("error out"=w276:errorcluster, "EncoderDevRef"=w277:T9)  [unwired: 5 in, 2 out]
              n149 = call <vilib>:"WPI_EncoderGet.vi"("error in (no error)"=w276, "EncoderDevRef"=w277) -> ("Distance"=w275:dbl)  [unwired: 4 in, 5 out]
              n150 = call <vilib>:"WPI_RobotDriveDelayAndUpdateSafety.vi"("Delay (s)"=0.1, "RobotDriveDevRef"=w323) -> ("RobotDriveDevRef 2"=w318:T16)  [unwired: 8 in, 1 out]
              n151 = Equal?(x=w275, y=100.0) -> (x = y?=w273:bool)
              n152 = case shown="True" w273 {
                tunnel: w318 -> [w346 w350]
                tunnel: [w346 w347] -> w320
                frame False {
                }
                frame True {
                  n153 = call-poly <vilib>:"WPI_RobotDriveArcadeDrive.vi"("Y axis value"=0.3, "X axis value"=0.0, "RobotDriveDevRef"=w350) -> ("RobotDriveDevRef"=w347:T16)  [unwired: 6 in, 2 out]
                }
              }
              n154 = call <vilib>:"WPI_DigitalInputOpen.vi"("DIO Channel"=w271) -> ("DigitalInputDevRef"=w268:T4)  [unwired: 1 in, 9 out]
              n155 = call <vilib>:"WPI_DigitalInputOpen.vi"("DIO Channel"=w272) -> ("DigitalInputDevRef"=w269:T4)  [unwired: 1 in, 9 out]
              n156 = call-poly <vilib>:"WPI_CounterToDigitalSource.vi"("DigitalInputDevRef"=w268) -> ("Digital Source"=w267:T5)  [unwired: 6 out]
              n157 = call-poly <vilib>:"WPI_CounterToDigitalSource.vi"("DigitalInputDevRef"=w269) -> ("Digital Source"=w270:T5)  [unwired: 6 out]
              n158 = call <vilib>:"WPI_EncoderOpen.vi"("DistancePerCount"=18.84955592153876, "BSource"=w270, "ASource"=w267) -> ("error out"=w264:errorcluster, "EncoderDevRef"=w265:T9)  [unwired: 5 in, 2 out]
              n159 = call <vilib>:"WPI_EncoderGet.vi"("error in (no error)"=w264, "EncoderDevRef"=w265) -> ("Distance"=w263:dbl)  [unwired: 4 in, 5 out]
              n160 = call <vilib>:"WPI_RobotDriveDelayAndUpdateSafety.vi"("Delay (s)"=0.1, "RobotDriveDevRef"=w320) -> ("RobotDriveDevRef 2"=w316:T16)  [unwired: 8 in, 1 out]
              n161 = Equal?(x=w263, y=100.0) -> (x = y?=w261:bool)
              n162 = case shown="True" w261 {
                tunnel: w316 -> [w341 w345]
                tunnel: [w341 w342] -> w317
                frame False {
                }
                frame True {
                  n163 = call-poly <vilib>:"WPI_RobotDriveArcadeDrive.vi"("Y axis value"=0.5, "X axis value"=0.0, "RobotDriveDevRef"=w345) -> ("RobotDriveDevRef"=w342:T16)  [unwired: 6 in, 2 out]
                }
              }
              n164 = call <vilib>:"WPI_DigitalInputOpen.vi"("DIO Channel"=w259) -> ("DigitalInputDevRef"=w256:T4)  [unwired: 1 in, 9 out]
              n165 = call <vilib>:"WPI_DigitalInputOpen.vi"("DIO Channel"=w260) -> ("DigitalInputDevRef"=w257:T4)  [unwired: 1 in, 9 out]
              n166 = call-poly <vilib>:"WPI_CounterToDigitalSource.vi"("DigitalInputDevRef"=w256) -> ("Digital Source"=w255:T5)  [unwired: 6 out]
              n167 = call-poly <vilib>:"WPI_CounterToDigitalSource.vi"("DigitalInputDevRef"=w257) -> ("Digital Source"=w258:T5)  [unwired: 6 out]
              n168 = call <vilib>:"WPI_EncoderOpen.vi"("DistancePerCount"=18.84955592153876, "BSource"=w258, "ASource"=w255) -> ("error out"=w252:errorcluster, "EncoderDevRef"=w253:T9)  [unwired: 5 in, 2 out]
              n169 = call <vilib>:"WPI_EncoderGet.vi"("error in (no error)"=w252, "EncoderDevRef"=w253) -> ("Distance"=w251:dbl)  [unwired: 4 in, 5 out]
              n170 = call <vilib>:"WPI_RobotDriveDelayAndUpdateSafety.vi"("Delay (s)"=0.1, "RobotDriveDevRef"=w317) -> ("RobotDriveDevRef 2"=w312:T16)  [unwired: 8 in, 1 out]
              n171 = Equal?(x=w251, y=100.0) -> (x = y?=w238:bool)
              n172 = case shown="True" w238 {
                tunnel: w312 -> [w336 w340]
                tunnel: [w336 w337] -> w313
                frame False {
                }
                frame True {
                  n173 = call-poly <vilib>:"WPI_RobotDriveArcadeDrive.vi"("Y axis value"=0.7, "X axis value"=0.0, "RobotDriveDevRef"=w340) -> ("RobotDriveDevRef"=w337:T16)  [unwired: 6 in, 2 out]
                }
              }
              n174 = call <vilib>:"WPI_DigitalInputOpen.vi"("DIO Channel"=w248) -> ("DigitalInputDevRef"=w245:T4)  [unwired: 1 in, 9 out]
              n175 = call <vilib>:"WPI_DigitalInputOpen.vi"("DIO Channel"=w249) -> ("DigitalInputDevRef"=w246:T4)  [unwired: 1 in, 9 out]
              n176 = call-poly <vilib>:"WPI_CounterToDigitalSource.vi"("DigitalInputDevRef"=w245) -> ("Digital Source"=w244:T5)  [unwired: 6 out]
              n177 = call-poly <vilib>:"WPI_CounterToDigitalSource.vi"("DigitalInputDevRef"=w246) -> ("Digital Source"=w247:T5)  [unwired: 6 out]
              n178 = call <vilib>:"WPI_EncoderOpen.vi"("DistancePerCount"=18.84955592153876, "BSource"=w247, "ASource"=w244) -> ("error out"=w241:errorcluster, "EncoderDevRef"=w242:T9)  [unwired: 5 in, 2 out]
              n179 = call <vilib>:"WPI_EncoderGet.vi"("error in (no error)"=w241, "EncoderDevRef"=w242) -> ("Distance"=w240:dbl)  [unwired: 4 in, 5 out]
              n180 = call <vilib>:"WPI_RobotDriveDelayAndUpdateSafety.vi"("Delay (s)"=0.1, "RobotDriveDevRef"=w313) -> ("RobotDriveDevRef 2"=w309:T16)  [unwired: 8 in, 1 out]
              n181 = Equal?(x=w240, y=100.0) -> (x = y?=w237:bool)
              n182 = case shown="True" w237 {
                tunnel: w309 -> [w331 w335]
                tunnel: [w331 w332] -> w310
                frame False {
                }
                frame True {
                  n183 = call-poly <vilib>:"WPI_RobotDriveArcadeDrive.vi"("Y axis value"=0.9, "X axis value"=0.0, "RobotDriveDevRef"=w335) -> ("RobotDriveDevRef"=w332:T16)  [unwired: 6 in, 2 out]
                }
              }
              n184 = call <vilib>:"WPI_DigitalInputOpen.vi"("DIO Channel"=w235) -> ("DigitalInputDevRef"=w232:T4)  [unwired: 1 in, 9 out]
              n185 = call <vilib>:"WPI_DigitalInputOpen.vi"("DIO Channel"=w236) -> ("DigitalInputDevRef"=w233:T4)  [unwired: 1 in, 9 out]
              n186 = call-poly <vilib>:"WPI_CounterToDigitalSource.vi"("DigitalInputDevRef"=w232) -> ("Digital Source"=w231:T5)  [unwired: 6 out]
              n187 = call-poly <vilib>:"WPI_CounterToDigitalSource.vi"("DigitalInputDevRef"=w233) -> ("Digital Source"=w234:T5)  [unwired: 6 out]
              n188 = call <vilib>:"WPI_EncoderOpen.vi"("DistancePerCount"=18.84955592153876, "BSource"=w234, "ASource"=w231) -> ("error out"=w228:errorcluster, "EncoderDevRef"=w229:T9)  [unwired: 5 in, 2 out]
              n189 = call <vilib>:"WPI_EncoderGet.vi"("error in (no error)"=w228, "EncoderDevRef"=w229) -> ("Distance"=w227:dbl)  [unwired: 4 in, 5 out]
              n190 = call <vilib>:"WPI_RobotDriveDelayAndUpdateSafety.vi"("Delay (s)"=0.1, "RobotDriveDevRef"=w310) -> ("RobotDriveDevRef 2"=w308:T16)  [unwired: 8 in, 1 out]
              n191 = Equal?(x=w227, y=100.0) -> (x = y?=w225:bool)
              n192 = case shown="True" w225 {
                tunnel: w308 -> [_ w330]
                frame False {
                }
                frame True {
                  n193 = call-poly <vilib>:"WPI_RobotDriveArcadeDrive.vi"("Y axis value"=0.5, "X axis value"=0.0, "RobotDriveDevRef"=w330) -> ()  [unwired: 6 in, 3 out]
                }
              }
            }
          }
        }
      }
    }
    frame Enabled {
    }
  }
  n194 = Index Array(array=w3, index #1=2 ("index")) -> ()  [unwired: 1 in, 2 out]
  n195 = call-poly <vilib>:"NT Write Value.vi"("Numeric Array"=w3, "Name"="Joystick 0/Axes") -> ()  [unwired: 9 in, 1 out]
